vi "Read Sentran Accuracy Test Settings.vi"(8 "error in (no error)":errorcluster, 11 "Boot Loader in":refnum<class "Boot Loader.lvclass">) -> (0 "error out":errorcluster, 2 "Sentran Accuracy Test Settings":T1 {"Max Moment (NM)" format="%.4f"; "Sample Time (s)" format="%.4f"; "Process Time (s)" format="%.4f"; "Force Tolerance (N)" format="%.4f"}, 3 "Boot Loader out":refnum<class "Boot Loader.lvclass">)   [LabVIEW 2016, in "Boot Loader.lvclass"]
uses:
  Boot Loader.lvclass
  Typedefs/SentranAccuracyTestSettings.ctl
  Settings/Settings.lvclass
  Typedefs/FAMT Typedefs.lvlib
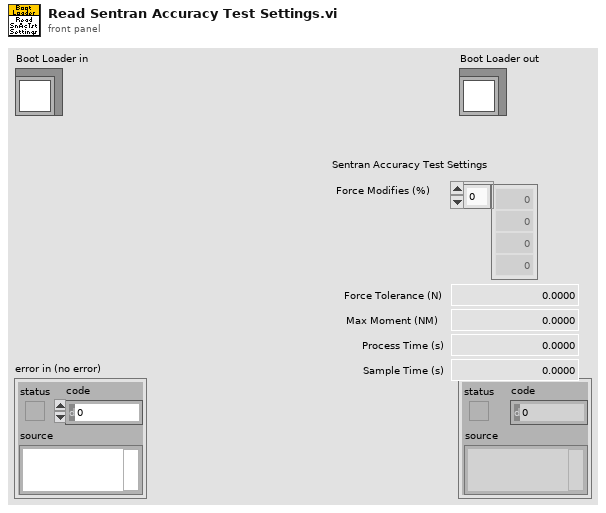
[diagram p1: front panel]
types:
  T1 = typedef "FAMT Typedefs.lvlib/SentranAccuracyTestSettings.ctl" = cluster{"Force Tolerance (N)":dbl, "Force Modifies (%)":dbl[], "Process Time (s)":dbl, "Sample Time (s)":dbl, "Max Moment (NM)":dbl}
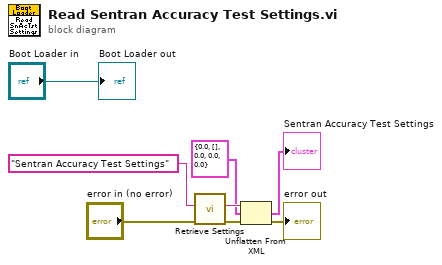
[diagram p0: block diagram]
diagram:
  n1 = call "Retrieve Settings.vi"("error in (no error)"="error in (no error)", "configName"="Sentran Accuracy Test Settings") -> ("error out"=w4:errorcluster, "xmlConfig"=w7:string)  [unwired: 7 in, 1 out]
  n2 = Unflatten From XML(xml string=w7, type=T1 {"Force Tolerance (N)"=0.0, "Force Modifies (%)"=[], "Process Time (s)"=0.0, "Sample Time (s)"=0.0, "Max Moment (NM)"=0.0} ("Sentran Accuracy Test Settings"), error in (no error)=w4) -> (value=→"Sentran Accuracy Test Settings":T1, error out=→"error out":errorcluster)
  "Boot Loader out" <- "Boot Loader in"
